vi "JanAssignmentZach.vi"() -> ()   [LabVIEW 2020]
uses:
  <vilib>/ULx/Create Channel.llb/ULx Create Channel (AI-Voltage-Basic).vi
  <vilib>/ULx/Timing.llb/ULx Timing (Sample Clock).vi
  <vilib>/ULx/Read.llb/ULx Read (Analog Wfm 1Chan NSamp).vi
panel:
  out "Elapsed Time (s)":dbl
  in  "Time Measurement Inerval (s)":dbl
  in  "Duration of Measurement (s)":dbl
  out "Waveform Graph":waveform(dbl)(graph)
  in  "samples per channel":i32=1000
  in  "rate":dbl=1000.0
  in  "physical channels":refnum<k21>
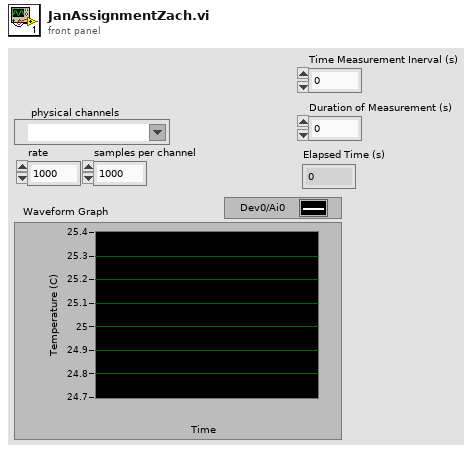
[diagram p1: front panel]
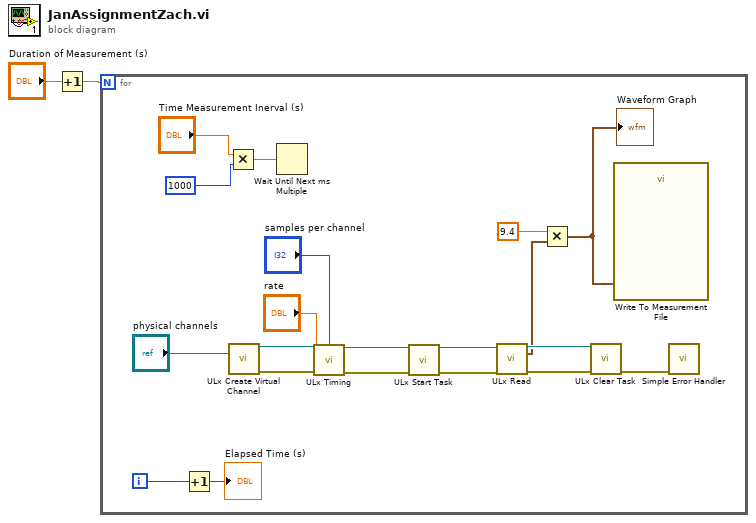
[diagram p0: block diagram]
diagram:
  n1 = Increment(x="Duration of Measurement (s)") -> (x+1=w2:dbl)
  n2 = for {
    N: w2 -> [_]
    i -> [w10]
    n3 = Increment(x=w10) -> (x+1=→"Elapsed Time (s)":i32)
    n4 = Multiply(x="Time Measurement Inerval (s)", y=1000) -> (x*y=w6:dbl)
    n5 = call-poly <vilib>:"ULx Create Virtual Channel.vi"("physical channels"="physical channels") -> ("task out"=w14:refnum<k24>, "error out"=w18:errorcluster)  [unwired: 13 in]
    n6 = Wait Until Next ms Multiple(millisecond multiple=w6) -> ()  [unwired: 1 out]
    n7 = call-poly <vilib>:"ULx Timing.vi"("task in"=w14, "samples per channel"="samples per channel", "rate"="rate", "error in"=w18) -> ("task out"=w15:refnum<k24>, "error out"=w19:errorcluster)  [unwired: 10 in]
    n8 = call <vilib>:"ULx Start Task.vi"("task in"=w15, "error in"=w19) -> ("task out"=w16:refnum<k24>, "error out"=w20:errorcluster)  [unwired: 12 in]
    n9 = call-poly <vilib>:"ULx Read.vi"("task in"=w16, "error in"=w20) -> ("task out"=w17:refnum<k24>, "data"=w5:waveform(dbl), "error out"=w21:errorcluster)  [unwired: 11 in]
    n10 = Multiply(x=9.4, y=w5) -> (x*y=w3:waveform(dbl))
    "Waveform Graph" <- w3
    n11 = call <vilib>:"ULx Clear Task.vi"("task in"=w17, "error in"=w21) -> ("error out"=w22:errorcluster)  [unwired: 13 in]
    n12 = call "Write To Measurement File"("Signals"=w3) -> ()  [unwired: 16 in, 3 out]
    n13 = call <vilib>:"Simple Error Handler.vi"("error in (no error)"=w22) -> ()  [unwired: 4 in, 5 out]
  }
